vi "Read Line Rate - Returns Default Value.vi"() -> ()   [LabVIEW 2017, in "Cobertura.Tests.lvlib" / "Coverage.lvlib"]
uses:
  Coverage.lvlib
  Cobertura/Coverage/Coverage.lvclass/Coverage.ctl
  Cobertura/Coverage/Read Line Rate.vi
  <vilib>/PNR/Transparent Assertions/Transparent Assertions/Transparent Assertions.lvlib
  Cobertura/Coverage/Coverage.lvclass
panel:
  out "error out":errorcluster
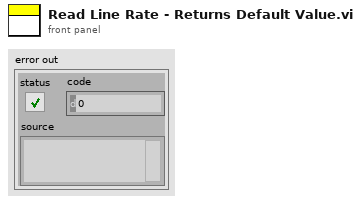
[diagram p1: front panel]
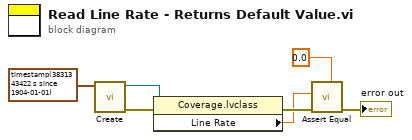
[diagram p0: block diagram]
diagram:
  n1 = call "Create.vi"("Timestamp"=timestamp(3831343422.3303647 s since 1904-01-01)) -> ("error out"=w1:errorcluster, "Coverage"=w2:refnum<class "Coverage.lvclass">)  [unwired: 9 in]
  n2 = property class="Coverage.lvclass"(reference=w2, error in=w1) -> (error out=w7:errorcluster, "Line Rate"=w5:dbl)  [unwired: 1 out]
  n3 = call <vilib>:"Assert Equal.vi"("Expected"=0.0 ("Branch Rate"), "error in (no error)"=w7, "Actual"=w5) -> ("error out"=→"error out":errorcluster)  [unwired: 8 in]
